vi "driveForwardSlow Command.vi"(5 "All Auto Drive constants":T1, 7 "Shifting controls":T5, 10 "Data":string[](array[string]), 11 "Robot dev revs":T6={"Drive"={"Drive Actuaters"={"Motor devRevs"={"Left Side Motors"={"Motor 1 devRev"={"DeviceStatus"={"status"=FALSE, "code"=0, "source"=""}, "Type"=enum."PWM", "PWM"={"Digital Module"=enum."Digital Module 1", "PWM Channel"=enum."PWM 1", "DeadBand"={"Name"="", "maxPositivePwm"=0, "minPositivePwm"=0, "centerPwm"=0, "maxNegativePwm"=0, "minNegativePwm"=0, "angularRange"=0}}, "CAN"={"Device Number"=0, "Control Mode"=enum."Percent VBus", "Semaphore"=refnum, "Max Vout"=0.0}, "Invert"=FALSE, "TransformRef"=refnum, "InvTransformRef"=refnum}, "Motor 2 devRev"={"DeviceStatus"={"status"=FALSE, "code"=0, "source"=""}, "Type"=enum."PWM", "PWM"={"Digital Module"=enum."Digital Module 1", "PWM Channel"=enum."PWM 1", "DeadBand"={"Name"="", "maxPositivePwm"=0, "minPositivePwm"=0, "centerPwm"=0, "maxNegativePwm"=0, "minNegativePwm"=0, "angularRange"=0}}, "CAN"={"Device Number"=0, "Control Mode"=enum."Percent VBus", "Semaphore"=refnum, "Max Vout"=0.0}, "Invert"=FALSE, "TransformRef"=refnum, "InvTransformRef"=refnum}, "Motor 3 devRev"={"DeviceStatus"={"status"=FALSE, "code"=0, "source"=""}, "Type"=enum."PWM", "PWM"={"Digital Module"=enum."Digital Module 1", "PWM Channel"=enum."PWM 1", "DeadBand"={"Name"="", "maxPositivePwm"=0, "minPositivePwm"=0, "centerPwm"=0, "maxNegativePwm"=0, "minNegativePwm"=0, "angularRange"=0}}, "CAN"={"Device Number"=0, "Control Mode"=enum."Percent VBus", "Semaphore"=refnum, "Max Vout"=0.0}, "Invert"=FALSE, "TransformRef"=refnum, "InvTransformRef"=refnum}}, "Right Side Motors"={"Motor 1 devRev"={"DeviceStatus"={"status"=FALSE, "code"=0, "source"=""}, "Type"=enum."PWM", "PWM"={"Digital Module"=enum."Digital Module 1", "PWM Channel"=enum."PWM 1", "DeadBand"={"Name"="", "maxPositivePwm"=0, "minPositivePwm"=0, "centerPwm"=0, "maxNegativePwm"=0, "minNegativePwm"=0, "angularRange"=0}}, "CAN"={"Device Number"=0, "Control Mode"=enum."Percent VBus", "Semaphore"=refnum, "Max Vout"=0.0}, "Invert"=FALSE, "TransformRef"=refnum, "InvTransformRef"=refnum}, "Motor 2 devRev"={"DeviceStatus"={"status"=FALSE, "code"=0, "source"=""}, "Type"=enum."PWM", "PWM"={"Digital Module"=enum."Digital Module 1", "PWM Channel"=enum."PWM 1", "DeadBand"={"Name"="", "maxPositivePwm"=0, "minPositivePwm"=0, "centerPwm"=0, "maxNegativePwm"=0, "minNegativePwm"=0, "angularRange"=0}}, "CAN"={"Device Number"=0, "Control Mode"=enum."Percent VBus", "Semaphore"=refnum, "Max Vout"=0.0}, "Invert"=FALSE, "TransformRef"=refnum, "InvTransformRef"=refnum}, "Motor 3 devRev"={"DeviceStatus"={"status"=FALSE, "code"=0, "source"=""}, "Type"=enum."PWM", "PWM"={"Digital Module"=enum."Digital Module 1", "PWM Channel"=enum."PWM 1", "DeadBand"={"Name"="", "maxPositivePwm"=0, "minPositivePwm"=0, "centerPwm"=0, "maxNegativePwm"=0, "minNegativePwm"=0, "angularRange"=0}}, "CAN"={"Device Number"=0, "Control Mode"=enum."Percent VBus", "Semaphore"=refnum, "Max Vout"=0.0}, "Invert"=FALSE, "TransformRef"=refnum, "InvTransformRef"=refnum}}, "dev Status"={"status"=FALSE, "code"=0, "source"=""}}, "SolenoidDevRef"={"DevStatus"={"status"=FALSE, "code"=0, "source"=""}, "Solenoid Module"=enum."Solenoid Module 1", "Forward Solenoid Channel"=enum."Solenoid 1", "Reverse Solenoid Channel"=enum."Solenoid 1"}}, "Drive Sensor data"={"Encoders"={"Right Encoder"={"DevStatus"={"status"=FALSE, "code"=0, "source"=""}, "EncoderIndex"=enum."Enc 0", "CounterIndex"=enum."Ctr 0", "DistancePerCount"=0.0, "Decoding Type"=enum."1x"}}, "GyroDevRef"={"DevStatus"={"status"=FALSE, "code"=0, "source"=""}, "Analog Module"=enum."Analog Module 1", "Analog Channel"=enum."AI 1", "Offset"=0.0, "Gain (VoltsPerDegree/Second)"=0.0}, "Last commanded Angle"=0.0}}, "Catapult devrevs"={"MotorControlDeviceRef"={"DeviceStatus"={"status"=FALSE, "code"=0, "source"=""}, "Type"=enum."PWM", "PWM"={"Digital Module"=enum."Digital Module 1", "PWM Channel"=enum."PWM 1", "DeadBand"={"Name"="", "maxPositivePwm"=0, "minPositivePwm"=0, "centerPwm"=0, "maxNegativePwm"=0, "minNegativePwm"=0, "angularRange"=0}}, "CAN"={"Device Number"=0, "Control Mode"=enum."Percent VBus", "Semaphore"=refnum, "Max Vout"=0.0}, "Invert"=FALSE, "TransformRef"=refnum, "InvTransformRef"=refnum}, "SolenoidDevRef"={"DevStatus"={"status"=FALSE, "code"=0, "source"=""}, "Solenoid Module"=enum."Solenoid Module 1", "Forward Solenoid Channel"=enum."Solenoid 1", "Reverse Solenoid Channel"=enum."Solenoid 1"}, "first limit switch"={"DevStatus"={"status"=FALSE, "code"=0, "source"=""}, "DIO Channel"=enum."DIO 1", "Digital Module"=enum."Digital Module 1"}, "second limit switch"={"DevStatus"={"status"=FALSE, "code"=0, "source"=""}, "DIO Channel"=enum."DIO 1", "Digital Module"=enum."Digital Module 1"}}, "Drive Joystick"={"Device"=enum."USB 1"}, "Operator Joystick"={"Device"=enum."USB 1"}, "roller devrevs"={"SolenoidDevRef"={"DevStatus"={"status"=FALSE, "code"=0, "source"=""}, "Solenoid Module"=enum."Solenoid Module 1", "Forward Solenoid Channel"=enum."Solenoid 1", "Reverse Solenoid Channel"=enum."Solenoid 1"}, "MotorControlDeviceRef"={"DeviceStatus"={"status"=FALSE, "code"=0, "source"=""}, "Type"=enum."PWM", "PWM"={"Digital Module"=enum."Digital Module 1", "PWM Channel"=enum."PWM 1", "DeadBand"={"Name"="", "maxPositivePwm"=0, "minPositivePwm"=0, "centerPwm"=0, "maxNegativePwm"=0, "minNegativePwm"=0, "angularRange"=0}}, "CAN"={"Device Number"=0, "Control Mode"=enum."Percent VBus", "Semaphore"=refnum, "Max Vout"=0.0}, "Invert"=FALSE, "TransformRef"=refnum, "InvTransformRef"=refnum}, "DigitalInputDevRef"={"DevStatus"={"status"=FALSE, "code"=0, "source"=""}, "DIO Channel"=enum."Invalid", "Digital Module"=enum."Digital Module 1"}}, "Puncher devrevs"={"SolenoidDevRef"={"DevStatus"={"status"=FALSE, "code"=0, "source"=""}, "Solenoid Module"=enum."Solenoid Module 1", "Forward Solenoid Channel"=enum."Solenoid 1", "Reverse Solenoid Channel"=enum."Solenoid 1"}, "DigitalInputDevRef"={"DevStatus"={"status"=FALSE, "code"=0, "source"=""}, "DIO Channel"=enum."DIO 1", "Digital Module"=enum."Digital Module 1"}}}) -> (3 "Robot dev revs out":T6={"Drive"={"Drive Actuaters"={"Motor devRevs"={"Left Side Motors"={"Motor 1 devRev"={"DeviceStatus"={"status"=FALSE, "code"=0, "source"=""}, "Type"=enum."PWM", "PWM"={"Digital Module"=enum."Digital Module 1", "PWM Channel"=enum."PWM 1", "DeadBand"={"Name"="", "maxPositivePwm"=0, "minPositivePwm"=0, "centerPwm"=0, "maxNegativePwm"=0, "minNegativePwm"=0, "angularRange"=0}}, "CAN"={"Device Number"=0, "Control Mode"=enum."Percent VBus", "Semaphore"=refnum, "Max Vout"=0.0}, "Invert"=FALSE, "TransformRef"=refnum, "InvTransformRef"=refnum}, "Motor 2 devRev"={"DeviceStatus"={"status"=FALSE, "code"=0, "source"=""}, "Type"=enum."PWM", "PWM"={"Digital Module"=enum."Digital Module 1", "PWM Channel"=enum."PWM 1", "DeadBand"={"Name"="", "maxPositivePwm"=0, "minPositivePwm"=0, "centerPwm"=0, "maxNegativePwm"=0, "minNegativePwm"=0, "angularRange"=0}}, "CAN"={"Device Number"=0, "Control Mode"=enum."Percent VBus", "Semaphore"=refnum, "Max Vout"=0.0}, "Invert"=FALSE, "TransformRef"=refnum, "InvTransformRef"=refnum}, "Motor 3 devRev"={"DeviceStatus"={"status"=FALSE, "code"=0, "source"=""}, "Type"=enum."PWM", "PWM"={"Digital Module"=enum."Digital Module 1", "PWM Channel"=enum."PWM 1", "DeadBand"={"Name"="", "maxPositivePwm"=0, "minPositivePwm"=0, "centerPwm"=0, "maxNegativePwm"=0, "minNegativePwm"=0, "angularRange"=0}}, "CAN"={"Device Number"=0, "Control Mode"=enum."Percent VBus", "Semaphore"=refnum, "Max Vout"=0.0}, "Invert"=FALSE, "TransformRef"=refnum, "InvTransformRef"=refnum}}, "Right Side Motors"={"Motor 1 devRev"={"DeviceStatus"={"status"=FALSE, "code"=0, "source"=""}, "Type"=enum."PWM", "PWM"={"Digital Module"=enum."Digital Module 1", "PWM Channel"=enum."PWM 1", "DeadBand"={"Name"="", "maxPositivePwm"=0, "minPositivePwm"=0, "centerPwm"=0, "maxNegativePwm"=0, "minNegativePwm"=0, "angularRange"=0}}, "CAN"={"Device Number"=0, "Control Mode"=enum."Percent VBus", "Semaphore"=refnum, "Max Vout"=0.0}, "Invert"=FALSE, "TransformRef"=refnum, "InvTransformRef"=refnum}, "Motor 2 devRev"={"DeviceStatus"={"status"=FALSE, "code"=0, "source"=""}, "Type"=enum."PWM", "PWM"={"Digital Module"=enum."Digital Module 1", "PWM Channel"=enum."PWM 1", "DeadBand"={"Name"="", "maxPositivePwm"=0, "minPositivePwm"=0, "centerPwm"=0, "maxNegativePwm"=0, "minNegativePwm"=0, "angularRange"=0}}, "CAN"={"Device Number"=0, "Control Mode"=enum."Percent VBus", "Semaphore"=refnum, "Max Vout"=0.0}, "Invert"=FALSE, "TransformRef"=refnum, "InvTransformRef"=refnum}, "Motor 3 devRev"={"DeviceStatus"={"status"=FALSE, "code"=0, "source"=""}, "Type"=enum."PWM", "PWM"={"Digital Module"=enum."Digital Module 1", "PWM Channel"=enum."PWM 1", "DeadBand"={"Name"="", "maxPositivePwm"=0, "minPositivePwm"=0, "centerPwm"=0, "maxNegativePwm"=0, "minNegativePwm"=0, "angularRange"=0}}, "CAN"={"Device Number"=0, "Control Mode"=enum."Percent VBus", "Semaphore"=refnum, "Max Vout"=0.0}, "Invert"=FALSE, "TransformRef"=refnum, "InvTransformRef"=refnum}}, "dev Status"={"status"=FALSE, "code"=0, "source"=""}}, "SolenoidDevRef"={"DevStatus"={"status"=FALSE, "code"=0, "source"=""}, "Solenoid Module"=enum."Solenoid Module 1", "Forward Solenoid Channel"=enum."Solenoid 1", "Reverse Solenoid Channel"=enum."Solenoid 1"}}, "Drive Sensor data"={"Encoders"={"Right Encoder"={"DevStatus"={"status"=FALSE, "code"=0, "source"=""}, "EncoderIndex"=enum."Enc 0", "CounterIndex"=enum."Ctr 0", "DistancePerCount"=0.0, "Decoding Type"=enum."1x"}}, "GyroDevRef"={"DevStatus"={"status"=FALSE, "code"=0, "source"=""}, "Analog Module"=enum."Analog Module 1", "Analog Channel"=enum."AI 1", "Offset"=0.0, "Gain (VoltsPerDegree/Second)"=0.0}, "Last commanded Angle"=0.0}}, "Catapult devrevs"={"MotorControlDeviceRef"={"DeviceStatus"={"status"=FALSE, "code"=0, "source"=""}, "Type"=enum."PWM", "PWM"={"Digital Module"=enum."Digital Module 1", "PWM Channel"=enum."PWM 1", "DeadBand"={"Name"="", "maxPositivePwm"=0, "minPositivePwm"=0, "centerPwm"=0, "maxNegativePwm"=0, "minNegativePwm"=0, "angularRange"=0}}, "CAN"={"Device Number"=0, "Control Mode"=enum."Percent VBus", "Semaphore"=refnum, "Max Vout"=0.0}, "Invert"=FALSE, "TransformRef"=refnum, "InvTransformRef"=refnum}, "SolenoidDevRef"={"DevStatus"={"status"=FALSE, "code"=0, "source"=""}, "Solenoid Module"=enum."Solenoid Module 1", "Forward Solenoid Channel"=enum."Solenoid 1", "Reverse Solenoid Channel"=enum."Solenoid 1"}, "first limit switch"={"DevStatus"={"status"=FALSE, "code"=0, "source"=""}, "DIO Channel"=enum."DIO 1", "Digital Module"=enum."Digital Module 1"}, "second limit switch"={"DevStatus"={"status"=FALSE, "code"=0, "source"=""}, "DIO Channel"=enum."DIO 1", "Digital Module"=enum."Digital Module 1"}}, "Drive Joystick"={"Device"=enum."USB 1"}, "Operator Joystick"={"Device"=enum."USB 1"}, "roller devrevs"={"SolenoidDevRef"={"DevStatus"={"status"=FALSE, "code"=0, "source"=""}, "Solenoid Module"=enum."Solenoid Module 1", "Forward Solenoid Channel"=enum."Solenoid 1", "Reverse Solenoid Channel"=enum."Solenoid 1"}, "MotorControlDeviceRef"={"DeviceStatus"={"status"=FALSE, "code"=0, "source"=""}, "Type"=enum."PWM", "PWM"={"Digital Module"=enum."Digital Module 1", "PWM Channel"=enum."PWM 1", "DeadBand"={"Name"="", "maxPositivePwm"=0, "minPositivePwm"=0, "centerPwm"=0, "maxNegativePwm"=0, "minNegativePwm"=0, "angularRange"=0}}, "CAN"={"Device Number"=0, "Control Mode"=enum."Percent VBus", "Semaphore"=refnum, "Max Vout"=0.0}, "Invert"=FALSE, "TransformRef"=refnum, "InvTransformRef"=refnum}, "DigitalInputDevRef"={"DevStatus"={"status"=FALSE, "code"=0, "source"=""}, "DIO Channel"=enum."Invalid", "Digital Module"=enum."Digital Module 1"}}, "Puncher devrevs"={"SolenoidDevRef"={"DevStatus"={"status"=FALSE, "code"=0, "source"=""}, "Solenoid Module"=enum."Solenoid Module 1", "Forward Solenoid Channel"=enum."Solenoid 1", "Reverse Solenoid Channel"=enum."Solenoid 1"}, "DigitalInputDevRef"={"DevStatus"={"status"=FALSE, "code"=0, "source"=""}, "DIO Channel"=enum."DIO 1", "Digital Module"=enum."Digital Module 1"}}})   [LabVIEW 2013]
uses:
  Robot dev revs.ctl
  Drive Code/Drive typedef.ctl
  Drive Code/Drive Motors Typedef.ctl
  Drive Code/GearBox Typedef.ctl
  <vilib>/Rock Robotics/WPI/MotorControl/WPI_MotorControlDeviceRef.ctl
  <vilib>/Rock Robotics/SystemInterfaces/Typedef/FPGA_TypedefDigitalModule.ctl
  <vilib>/Rock Robotics/SystemInterfaces/DIO/FPGA_DIOPWMChannel.ctl
  <vilib>/Rock Robotics/WPI/PWM/WPI_PWMDeadband.ctl
  <vilib>/Rock Robotics/WPI/CAN/Jaguar/SubVIs/WPI_CANJaguar_ControlMode.ctl
  <vilib>/Rock Robotics/WPI/PWM/WPI_PWMTransform_ConPane.ctl
  <vilib>/Rock Robotics/WPI/Solenoid/WPI_SolenoidDevRef.ctl
  <vilib>/Rock Robotics/SystemInterfaces/Typedef/FPGA_TypedefSolenoidModule.ctl
  <vilib>/Rock Robotics/WPI/Solenoid/WPI_SolenoidChannel.ctl
  Drive Code/Drive Sensor Typedef.ctl
  <vilib>/Rock Robotics/WPI/Encoder/WPI_EncoderDevRef.ctl
  <vilib>/Rock Robotics/SystemInterfaces/Encoder/FPGA_EncoderIdx.ctl
  <vilib>/Rock Robotics/SystemInterfaces/Counter/FPGA_CounterCtrSystemIndex.ctl
  <vilib>/Rock Robotics/WPI/Encoder/WPI_EncoderType.ctl
  <vilib>/Rock Robotics/WPI/Gyro/WPI_GyroDevRef.ctl
  <vilib>/Rock Robotics/SystemInterfaces/Typedef/FPGA_TypedefAnalogModule.ctl
  <vilib>/Rock Robotics/SystemInterfaces/AI/FPGA_AIChannel.ctl
  catapult code/catapult type def.ctl
  <vilib>/Rock Robotics/WPI/DigitalInput/WPI_DigitalInputDevRef.ctl
  <vilib>/Rock Robotics/SystemInterfaces/DIO/FPGA_DIOChannel.ctl
  <vilib>/Rock Robotics/WPI/Joystick/WPI_JoystickDevRef.ctl
  <vilib>/Rock Robotics/WPI/Joystick/WPI_JoystickDeviceEnum.ctl
  Roller V2/roller typedef.ctl
  Puncher/Puncher type.ctl
  Drive Auto/All Auto Drive constants.ctl
  Drive Auto/Drive auto constants.ctl
  Drive Code/Auto Transmission Code/All Shifter Constants.ctl
  Drive Code/Auto Transmission Code/Shift Constants.ctl
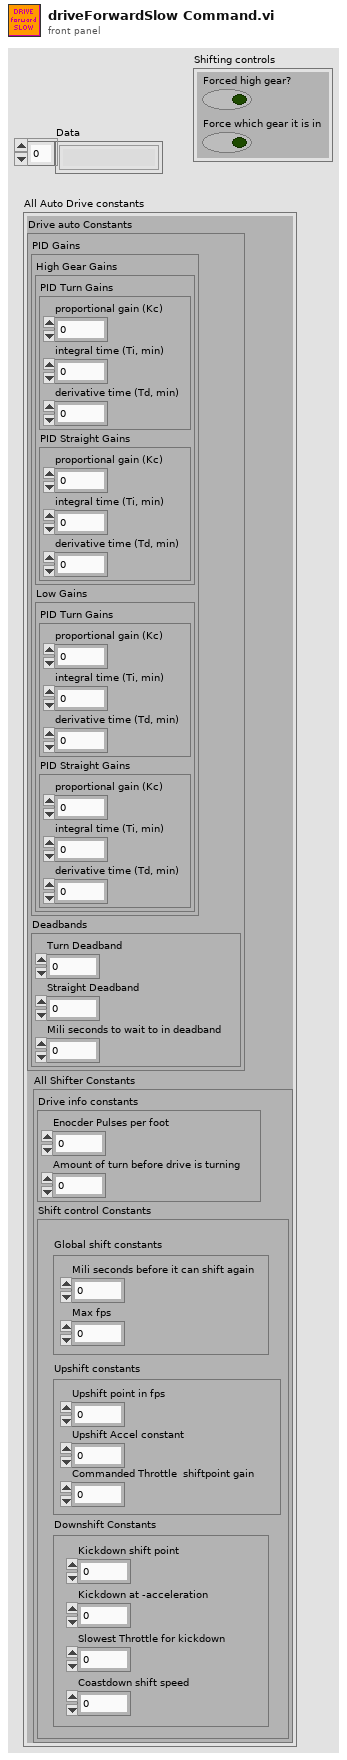
[diagram p1: front panel]
types:
  T1 = typedef "All Auto Drive constants.ctl" = cluster{"Drive auto Constants":T2, "All Shifter Constants":T3}
  T2 = typedef "Drive auto constants.ctl" = cluster{"PID Gains":cluster{"High Gear Gains":cluster{"PID Turn Gains":cluster{"proportional gain (Kc)":dbl, "integral time (Ti, min)":dbl, "derivative time (Td, min)":dbl}, "PID Straight Gains":cluster{"proportional gain (Kc)":dbl, "integral time (Ti, min)":dbl, "derivative time (Td, min)":dbl}}, "Low Gains":cluster{"PID Turn Gains":cluster{"proportional gain (Kc)":dbl, "integral time (Ti, min)":dbl, "derivative time (Td, min)":dbl}, "PID Straight Gains":cluster{"proportional gain (Kc)":dbl, "integral time (Ti, min)":dbl, "derivative time (Td, min)":dbl}}}, "Deadbands":cluster{"Turn Deadband":dbl, "Straight Deadband":dbl, "Mili seconds to wait to in deadband":u32}}
  T3 = typedef "All Shifter Constants.ctl" = cluster{"Drive info constants":cluster{"Enocder Pulses per foot":dbl, "Amount of turn before drive is turning":dbl}, "Shift control Constants":T4}
  T4 = typedef "Shift Constants.ctl" = cluster{"Global shift constants":cluster{"Mili seconds before it can shift again":u32, "Max fps":dbl}, "Upshift constants":cluster{"Upshift point in fps":dbl, "Upshift Accel constant":dbl, "Commanded Throttle  shiftpoint gain":dbl}, "Downshift Constants":cluster{"Kickdown shift point":dbl, "Kickdown at -acceleration":dbl, "Slowest Throttle for kickdown":dbl, "Coastdown shift speed":dbl}}
  T5 = cluster{"Forced high gear?":bool, "Force which gear it is in":bool}
  T6 = typedef "Robot dev revs.ctl" = cluster{"Drive":T7, "Catapult devrevs":T28, "Drive Joystick":T31, "Operator Joystick":T31, "roller devrevs":T33, "Puncher devrevs":T34}
  T7 = typedef "Drive typedef.ctl" = cluster{"Drive Actuaters":cluster{"Motor devRevs":T8, "SolenoidDevRef":T17}, "Drive Sensor data":T20}
  T8 = typedef "Drive Motors Typedef.ctl" = cluster{"Left Side Motors":T9, "Right Side Motors":T9, "dev Status":errorcluster}
  T9 = typedef "GearBox Typedef.ctl" = cluster{"Motor 1 devRev":T10, "Motor 2 devRev":T10, "Motor 3 devRev":T10}
  T10 = typedef "WPI_MotorControlDeviceRef.ctl" = cluster{"DeviceStatus":errorcluster, "Type":enum16{"PWM", "CAN"}, "PWM":cluster{"Digital Module":T11, "PWM Channel":T12, "DeadBand":T13}, "CAN":cluster{"Device Number":u8, "Control Mode":T14, "Semaphore":T15, "Max Vout":dbl}, "Invert":bool, "TransformRef":T16, "InvTransformRef":T16}
  T11 = typedef "FPGA_TypedefDigitalModule.ctl" = enum16{"Digital Module 1", "Digital Module 2"}
  T12 = typedef "FPGA_DIOPWMChannel.ctl" = enum8{"PWM 1", "PWM 2", "PWM 3", "PWM 4", "PWM 5", "PWM 6", "PWM 7", "PWM 8", "PWM 9", "PWM 10", "Invalid"}
  T13 = typedef "WPI_PWMDeadband.ctl" = cluster{"Name":string, "maxPositivePwm":i32, "minPositivePwm":i32, "centerPwm":i32, "maxNegativePwm":i32, "minNegativePwm":i32, "angularRange":u16}
  T14 = typedef "WPI_CANJaguar_ControlMode.ctl" = enum8{"Percent VBus", "Current", "Speed", "Position", "Voltage"}
  T15 = typedef "Semaphore RefNum" = refnum<k1>
  T16 = typedef "WPI_PWMTransform_ConPane.ctl" = refnum<vi>
  T17 = typedef "WPI_SolenoidDevRef.ctl" = cluster{"DevStatus":errorcluster, "Solenoid Module":T18, "Forward Solenoid Channel":T19, "Reverse Solenoid Channel":T19}
  T18 = typedef "FPGA_TypedefSolenoidModule.ctl" = enum16{"Solenoid Module 1", "Solenoid Module 2"}
  T19 = typedef "WPI_SolenoidChannel.ctl" = enum8{"Solenoid 1", "Solenoid 2", "Solenoid 3", "Solenoid 4", "Solenoid 5", "Solenoid 6", "Solenoid 7", "Solenoid 8", "Invalid"}
  T20 = typedef "Drive Sensor Typedef.ctl" = cluster{"Encoders":cluster{"Right Encoder":T21}, "GyroDevRef":T25, "Last commanded Angle":dbl}
  T21 = typedef "WPI_EncoderDevRef.ctl" = cluster{"DevStatus":errorcluster, "EncoderIndex":T22, "CounterIndex":T23, "DistancePerCount":dbl, "Decoding Type":T24}
  T22 = typedef "FPGA_EncoderIdx.ctl" = enum8{"Enc 0", "Enc 1", "Enc 2", "Enc 3", "Invalid"}
  T23 = typedef "FPGA_CounterCtrSystemIndex.ctl" = enum8{"Ctr 0", "Ctr 1", "Ctr 2", "Ctr 3", "Ctr 4", "Ctr 5", "Ctr 6", "Ctr 7", "Invalid"}
  T24 = typedef "WPI_EncoderType.ctl" = enum16{"1x", "2x", "4x"}
  T25 = typedef "WPI_GyroDevRef.ctl" = cluster{"DevStatus":errorcluster, "Analog Module":T26, "Analog Channel":T27, "Offset":dbl, "Gain (VoltsPerDegree/Second)":dbl}
  T26 = typedef "FPGA_TypedefAnalogModule.ctl" = enum16{"Analog Module 1", "Analog Module 2"}
  T27 = typedef "FPGA_AIChannel.ctl" = enum8{"AI 1", "AI 2", "AI 3", "AI 4", "AI 5", "AI 6", "AI 7", "AI 8", "Invalid"}
  T28 = typedef "catapult type def.ctl" = cluster{"MotorControlDeviceRef":T10, "SolenoidDevRef":T17, "first limit switch":T29, "second limit switch":T29}
  T29 = typedef "WPI_DigitalInputDevRef.ctl" = cluster{"DevStatus":errorcluster, "DIO Channel":T30, "Digital Module":T11}
  T30 = typedef "FPGA_DIOChannel.ctl" = enum8{"DIO 1", "DIO 2", "DIO 3", "DIO 4", "DIO 5", "DIO 6", "DIO 7", "DIO 8", "DIO 9", "DIO 10", "DIO 11", "DIO 12", "DIO 13", "DIO 14", "Invalid"}
  T31 = typedef "WPI_JoystickDevRef.ctl" = cluster{"Device":T32}
  T32 = typedef "WPI_JoystickDeviceEnum.ctl" = enum16{"USB 1", "USB 2", "USB 3", "USB 4", "Kinect 1", "Kinect 2"}
  T33 = typedef "roller typedef.ctl" = cluster{"SolenoidDevRef":T17, "MotorControlDeviceRef":T10, "DigitalInputDevRef":T29}
  T34 = typedef "Puncher type.ctl" = cluster{"SolenoidDevRef":T17, "DigitalInputDevRef":T29}
  T35 = cluster{"Setpoint Angle":dbl, "Setpoint Distance":dbl}
  T36 = cluster{"Turn Speed Limits":cluster{"upper limit":dbl, "lower limit":dbl}, "Straight Speed Limits":cluster{"upper limit":dbl, "lower limit":dbl}}
  T37 = cluster{"High Gear Gains":cluster{"PID Turn Gains":cluster{"proportional gain (Kc)":dbl, "integral time (Ti, min)":dbl, "derivative time (Td, min)":dbl}, "PID Straight Gains":cluster{"proportional gain (Kc)":dbl, "integral time (Ti, min)":dbl, "derivative time (Td, min)":dbl}}, "Low Gains":cluster{"PID Turn Gains":cluster{"proportional gain (Kc)":dbl, "integral time (Ti, min)":dbl, "derivative time (Td, min)":dbl}, "PID Straight Gains":cluster{"proportional gain (Kc)":dbl, "integral time (Ti, min)":dbl, "derivative time (Td, min)":dbl}}}
  T38 = cluster{"Turn Deadband":dbl, "Straight Deadband":dbl, "Mili seconds to wait to in deadband":u32}
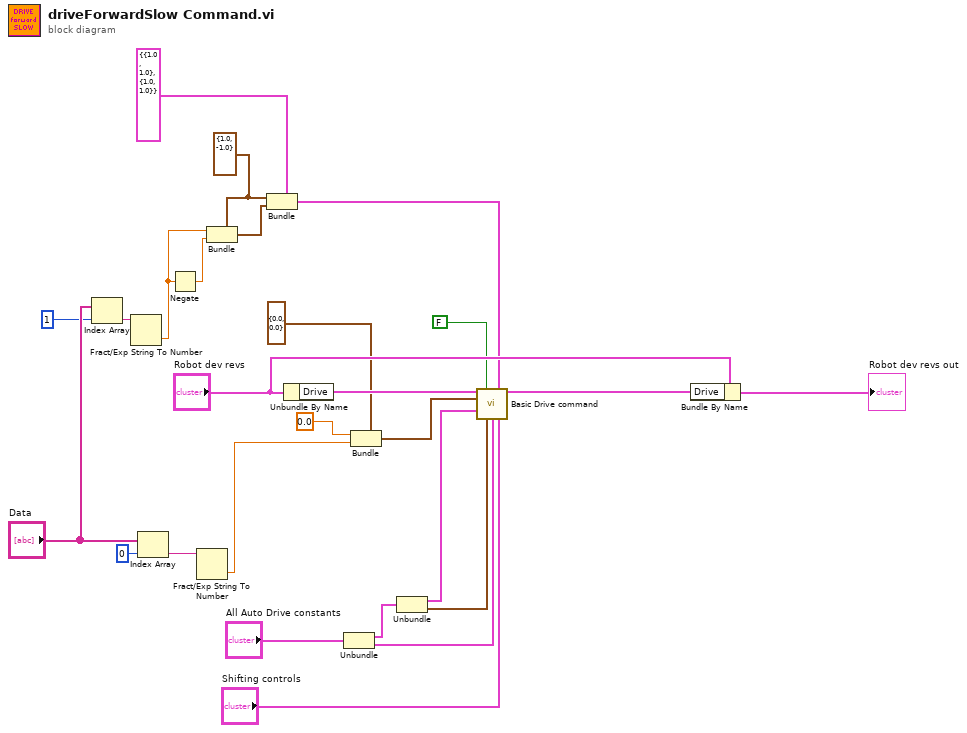
[diagram p0: block diagram]
diagram:
  w6 = cluster{"upper limit":dbl, "lower limit":dbl} {"upper limit"=1.0, "lower limit"=-1.0} ("Turn Speed Limits")
  n1 = Index Array(array="Data", index=1) -> (element=w3:string)
  n2 = Fract/Exp String To Number(string=w3) -> (number=w2:dbl)  [unwired: 3 in, 1 out]
  n3 = Index Array(array="Data", index=0) -> (element=w18:string)
  n4 = Negate(x=w2) -> (-x=w4:dbl)
  n5 = Fract/Exp String To Number(string=w18) -> (number=w17:dbl)  [unwired: 3 in, 1 out]
  n6 = Bundle(cluster=w6, "upper limit"=w2, "lower limit"=w4) -> (w5:cluster{"upper limit":dbl, "lower limit":dbl})
  n7 = Bundle(cluster=T36 {"Turn Speed Limits"={"upper limit"=1.0, "lower limit"=1.0}, "Straight Speed Limits"={"upper limit"=1.0, "lower limit"=1.0}} ("Speed Limits"), "Turn Speed Limits"=w6, "Straight Speed Limits"=w5) -> (w1:T36)
  n8 = Unbundle By Name("Robot dev revs") -> ("Drive"=w26:T7)
  n9 = Unbundle("All Auto Drive constants") -> ("Drive auto Constants"=w15:T2, "All Shifter Constants"=w12:T3)
  n10 = Bundle(cluster=T35 {"Setpoint Angle"=0.0, "Setpoint Distance"=0.0} ("Setpoints"), "Setpoint Angle"=0.0, "Setpoint Distance"=w17) -> (w21:T35)
  n11 = Unbundle(w15) -> ("PID Gains"=w14:T37, "Deadbands"=w13:T38)
  n12 = call "Basic Drive command.vi"("Drive"=w26, "Turn Only?"=FALSE, "Speed Limits"=w1, "Setpoints"=w21, "PID Gains"=w14, "Deadbands"=w13, "All Shifter Constants"=w12, "Shifting controls"="Shifting controls") -> ("Drive out"=w24:T7)  [unwired: 6 in, 1 out]
  n13 = Bundle By Name(cluster="Robot dev revs", "Drive"=w24) -> (→"Robot dev revs out":T6)
